vi "UMLEditor CreateNoteText.vi"(1 "graph":refnum<class "Graph.lvclass">, 2 "NoteEdge?":refnum<class "AbstractEdge.lvclass">, 5 "error in (no error)":errorcluster) -> (19 "error out":errorcluster)   [LabVIEW 2016]
doc: "Gets current diagram values"
uses:
  <resource>/Framework/Providers/Open_GDS/UML/Graph_class/Graph.lvclass
  <resource>/Framework/Providers/Open_GDS/UML/AbstractEdge_class/AbstractEdge.lvclass
  <resource>/Framework/Providers/Open_GDS/UML/General/Point/Point Point2D.ctl
  <resource>/Framework/Providers/Open_GDS/UML/AbstractNode_class/AbstractNode.lvclass
  <resource>/Framework/Providers/Open_GDS/UML/NoteNode_class/NoteNode.lvclass
  <resource>/Framework/Providers/Open_GDS/UML/MultiLineString_class/MultiLineString.lvclass
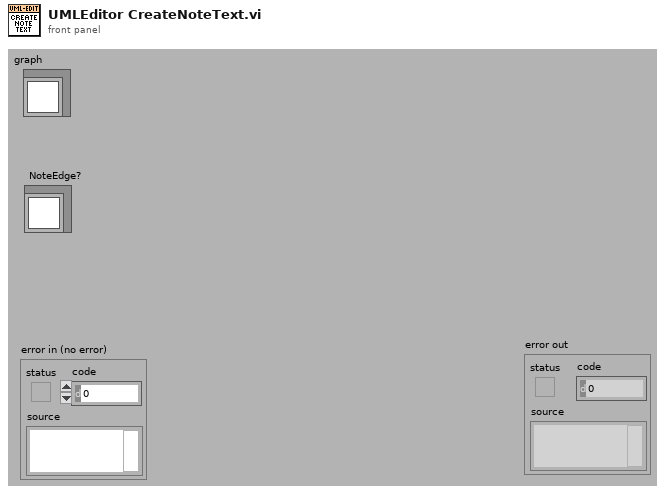
[diagram p1: front panel]
types:
  T1 = typedef "Point Point2D.ctl" = cluster{"x":dbl, "y":dbl}
  T2 = cluster{"text":string, "empty picture":picture, string}
  T3 = typedef "Rectangle Rectangle2D.ctl" = cluster{"x":dbl, "y":dbl, "width":dbl, "height":dbl}
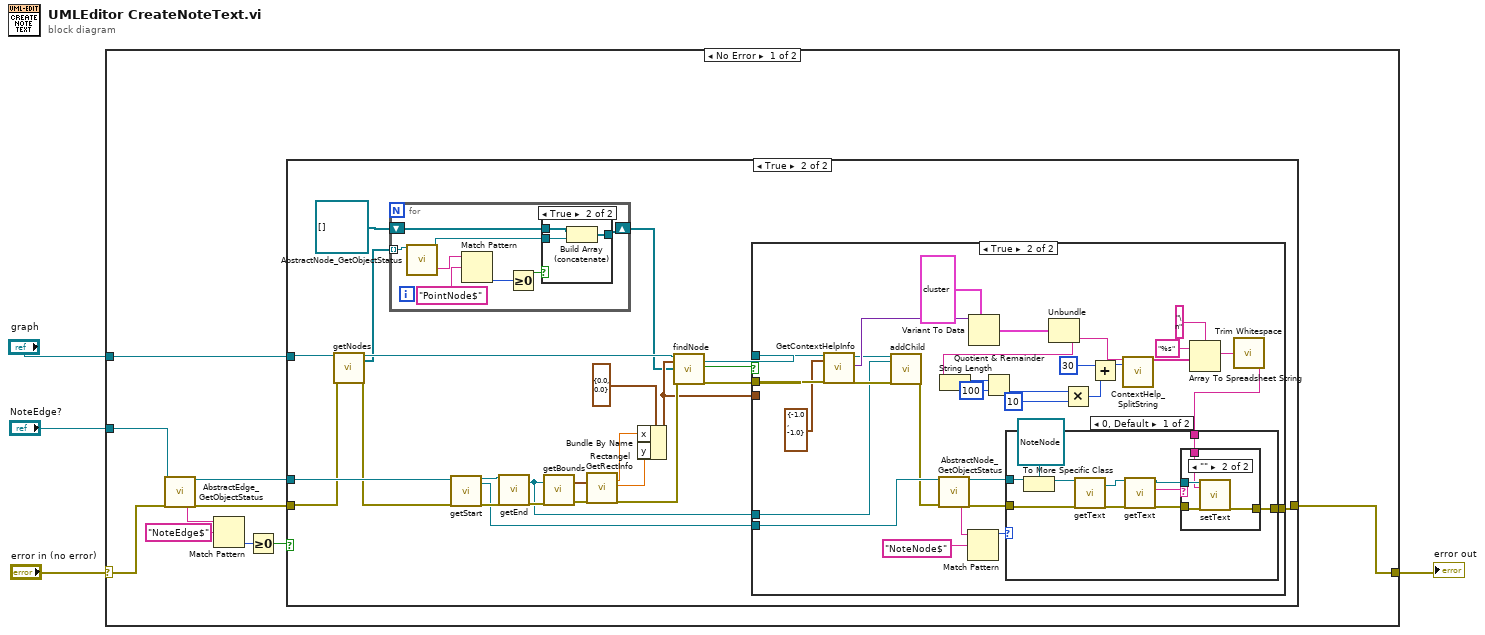
[diagram p0: block diagram]
diagram:
  n1 = case shown="No Error" "error in (no error)" {
    selector: "error in (no error)" -> [w8 w100]
    tunnel: [w7 w100] -> w3
    tunnel: "NoteEdge?" -> [w10 _]
    tunnel: "graph" -> [w6 _]
    frame No Error {
      n2 = call <resource>:"AbstractEdge_GetObjectStatus.vi"("reference in"=w10, "error in (no error)"=w8) -> ("Class name"=w13:string, "reference out"=w5:refnum<class "AbstractEdge.lvclass">, "error out"=w14:errorcluster)  [unwired: 9 in, 6 out]
      n3 = Match Pattern(string=w13, regular expression="NoteEdge$") -> (offset past match=w11:i32)  [unwired: 4 out]
      n4 = Greater Or Equal To 0?(x=w11) -> (x >= 0?=w9:bool)
      n5 = case shown="True" w9 {
        tunnel: w14 -> [w15 w26]
        tunnel: [w15 w21] -> w7
        tunnel: w6 -> [_ w28]
        tunnel: w5 -> [_ w38]
        frame False {
        }
        frame True {
          n6 = call-dynamic "getNodes.vi"("reference"=w28, "error in (no error)"=w26) -> ("reference out"=w27:refnum<class "Graph.lvclass">, "nodes"=w24:refnum<class "AbstractNode.lvclass">[], "error out"=w25:errorcluster)  [unwired: 15 in]
          n7 = for {
            tunnel: w24 -> [w45] mode=indexing
            shift-right: [w40] -> w17
            shift-left: refnum<class "AbstractNode.lvclass">[] [] -> [w42]
            n8 = call <resource>:"AbstractNode_GetObjectStatus.vi"("reference in"=w45) -> ("Class name"=w44:string, "reference out"=w41:refnum<class "AbstractNode.lvclass">)  [unwired: 1 in, 16 out]
            n9 = Match Pattern(string=w44, regular expression="PointNode$") -> (offset past match=w47:i32)  [unwired: 4 out]
            n10 = Greater Or Equal To 0?(x=w47) -> (x >= 0?=w43:bool)
            n11 = case shown="True" w43 {
              tunnel: w42 -> [w48 w51]
              tunnel: w41 -> [_ w50]
              tunnel: [w48 w49] -> w40
              frame False {
              }
              frame True {
                n12 = Build Array (concatenate)(w51, w50) -> (w49:refnum<class "AbstractNode.lvclass">[])
              }
            }
          }
          n13 = call-dynamic "getStart.vi"("reference"=w38, "error in (no error)"=w25) -> ("reference out"=w37:refnum<class "AbstractEdge.lvclass">, "startNode"=w20:refnum<class "AbstractNode.lvclass">, "error out"=w39:errorcluster)  [unwired: 14 in, 1 out]
          n14 = call-dynamic "getEnd.vi"("reference"=w37, "error in (no error)"=w39) -> ("endNode"=w18:refnum<class "AbstractNode.lvclass">, "error out"=w36:errorcluster)  [unwired: 14 in, 2 out]
          n15 = call-dynamic "getBounds.vi"("reference"=w18, "error in (no error)"=w36) -> ("bounds"=w35:T3, "error out"=w34:errorcluster)  [unwired: 15 in, 1 out]
          n16 = call <resource>:"Rectangel GetRectInfo.vi"("bounds"=w35, "error in (no error)"=w34) -> ("centerX"=w23:dbl, "centerY"=w22:dbl, "error out"=w32:errorcluster)  [unwired: 15 out]
          n17 = Bundle By Name(cluster=T1 {"x"=0.0, "y"=0.0} ("point2D"), "x"=w23, "y"=w22) -> (w29:T1)
          n18 = call-dynamic "findNode.vi"("reference"=w27, "point2D"=w29, "IgnoreTheseNodes"=w17, "error in (no error)"=w32) -> ("node"=w31:refnum<class "AbstractNode.lvclass">, "found"=w19:bool, "error out"=w30:errorcluster)  [unwired: 12 in, 1 out]
          n19 = case shown="True" w19 {
            tunnel: w31 -> [_ w82]
            tunnel: w30 -> [w52 w81]
            tunnel: w29 -> [_ _]
            tunnel: [w52 w72] -> w21
            tunnel: w20 -> [_ w71]
            tunnel: w18 -> [_ w67]
            frame False {
            }
            frame True {
              n20 = call-dynamic "GetContextHelpInfo.vi"("reference"=w82, "MousePos"=T1 {"x"=-1.0, "y"=-1.0}, "error in (no error)"=w81) -> ("reference out"=w70:refnum<class "AbstractNode.lvclass">, "ContextHelpInfo"=w80:variant, "error out"=w69:errorcluster)  [unwired: 13 in, 1 out]
              n21 = call-dynamic "addChild.vi"("reference"=w70, "node"=w67, "error in (no error)"=w69) -> ("error out"=w68:errorcluster)  [unwired: 15 in, 1 out]
              n22 = call <resource>:"AbstractNode_GetObjectStatus.vi"("reference in"=w71, "error in (no error)"=w68) -> ("Class name"=w76:string, "reference out"=w73:refnum<class "AbstractNode.lvclass">, "error out"=w74:errorcluster)  [unwired: 15 out]
              n23 = Match Pattern(string=w76, regular expression="NoteNode$") -> (offset past match=w75:i32)  [unwired: 4 out]
              n24 = Variant To Data(type=T2 {"text"="", "empty picture"=bytes[0], ""} ("output cluster"), Variant=w80) -> (data=w78:T2)  [unwired: 1 in, 1 out]
              n25 = Unbundle(w78) -> (w61:string)  [unwired: 2 out]
              n26 = String Length(string=w61) -> (length=w60:i32)
              n27 = Quotient & Remainder(x=w60, y=100) -> (floor(x/y)=w56:i32)  [unwired: 1 out]
              n28 = Multiply(x=w56, y=10) -> (x*y=w54:i32)
              n29 = Add(x=30, y=w54) -> (x+y=w58:i32)
              n30 = call <resource>:"ContextHelp_SplitString.vi"("string"=w61, "Max string length"=w58) -> ("Array"=w66:string[])  [unwired: 17 out]
              n31 = Array To Spreadsheet String(delimiter (Tab)="\n", array=w66, 3:"%s" ("format string")) -> (spreadsheet string=w63:string)
              n32 = call <vilib>:"Trim Whitespace.vi"("string"=w63) -> ("trimmed string"=w62:string)  [unwired: 1 in]
              n33 = case shown="0, Default" w75 {
                tunnel: w74 -> [w93 w99]
                tunnel: w73 -> [w84 _]
                tunnel: [w88 w99] -> w72
                tunnel: w62 -> [w87 _]
                frame 0, Default {
                  n34 = To More Specific Class(target class=refnum<class "NoteNode.lvclass"> refnum ("reference"), reference=w84) -> (specific class reference=w83:refnum<class "NoteNode.lvclass">)  [unwired: 1 in, 1 out]
                  n35 = call-dynamic "getText.vi"("reference"=w83, "error in (no error)"=w93) -> ("text"=w86:refnum<class "MultiLineString.lvclass">, "error out"=w92:errorcluster)  [unwired: 15 in, 1 out]
                  n36 = call-dynamic "getText.vi"("reference"=w86, "error in (no error)"=w92) -> ("reference out"=w89:refnum<class "MultiLineString.lvclass">, "text"=w91:string, "error out"=w90:errorcluster)  [unwired: 15 in]
                  n37 = case shown="\"\"" w91 {
                    tunnel: w90 -> [w94 w98]
                    tunnel: w89 -> [_ w97]
                    tunnel: [w94 w96] -> w88
                    tunnel: w87 -> [_ w95]
                    frame "False", Default {
                    }
                    frame "" {
                      n38 = call-dynamic "setText.vi"("reference"=w97, "text"=w95, "error in (no error)"=w98) -> ("error out"=w96:errorcluster)  [unwired: 15 in, 1 out]
                    }
                  }
                }
                frame -1 {
                }
              }
            }
          }
        }
      }
    }
    frame Error {
    }
  }
  "error out" <- w3
